vi "No Op.vi"(7 "Sender":refnum<class "Sender.lvclass">, 11 "No Op in":refnum<class "No Op.lvclass">) -> (3 "No Op out":refnum<class "No Op.lvclass">)   [LabVIEW 2020, in "jettl.lvlib" / "No Op Msg.lvlib" / "No Op.lvclass"]
uses:
  No Op.lvclass
  Sender/Sender/Sender.lvclass
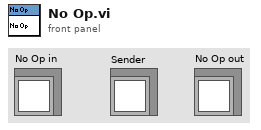
[diagram p1: front panel]
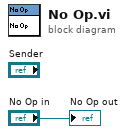
[diagram p0: block diagram]
diagram:
  "No Op out" <- "No Op in"
